vi "Trim.vi"(10 "String":string) -> (2 "TrimStr":string)   [LabVIEW 2013]
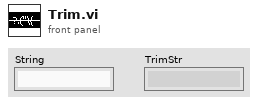
[diagram p1: front panel]
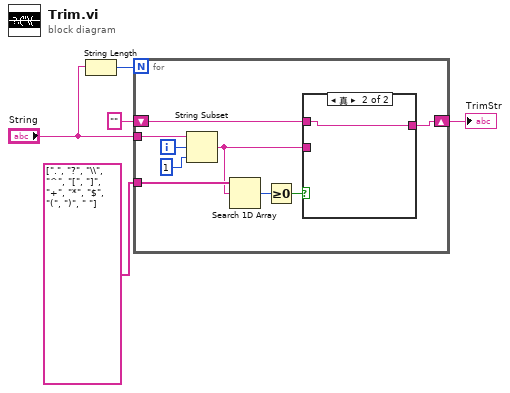
[diagram p0: block diagram]
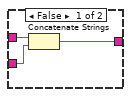
[diagram p2: hidden frame]
diagram:
  n1 = String Length(string="String") -> (length=w4:i32)
  n2 = for {
    N: w4 -> [_]
    tunnel: "String" -> [w14]
    tunnel: string[] [".", "?", "\\", "^", "[", "]", "+", "*", "$", "(", ")", " "] ("一维数组") -> [w11]
    shift-right: [w9] -> w5
    shift-left: "" -> [w8]
    i -> [w13]
    n3 = String Subset(string=w14, offset (0)=w13, length (rest)=1 ("长度（剩余）")) -> (substring=w6:string)
    n4 = Search 1D Array(1D array=w11, element=w6) -> (index of element=w10:i32)  [unwired: 1 in]
    n5 = Greater Or Equal To 0?(x=w10) -> (x >= 0?=w7:bool)
    n6 = case shown="真" w7 {
      tunnel: [w15 w18] -> w9
      tunnel: w8 -> [w17 w18]
      tunnel: w6 -> [w16 _]
      frame False {
        n7 = Concatenate Strings(w17, w16) -> (w15:string)
      }
      frame True {
      }
    }
  }
  "TrimStr" <- w5
